vi "Elevator Controller.vi"(8 "error in (no error)":errorcluster, 11 "View Model":T1) -> (0 "error out":errorcluster)   [LabVIEW 2017]
doc: "Handles all elevator operations."
uses:
  View Model/Controls/View Model.ctl
  Error Handler/Controls/Error Model.ctl
  Error Handler/Controls/Error EventData.ctl
  Error Handler/Controls/Error Type.ctl
  Controls/Elevator Model.ctl
  Controls/Elevator Overhead.ctl
  Controls/Elevator States.ctl
  Controls/Elevator Location.ctl
  Controls/Elevator Command Event.ctl
  Controls/Elevator Commands.ctl
  Configuration/Controls/Configuration Model.ctl
  Configuration/Controls/Configuration Data.ctl
  View Model/Controls/Shared Model.ctl
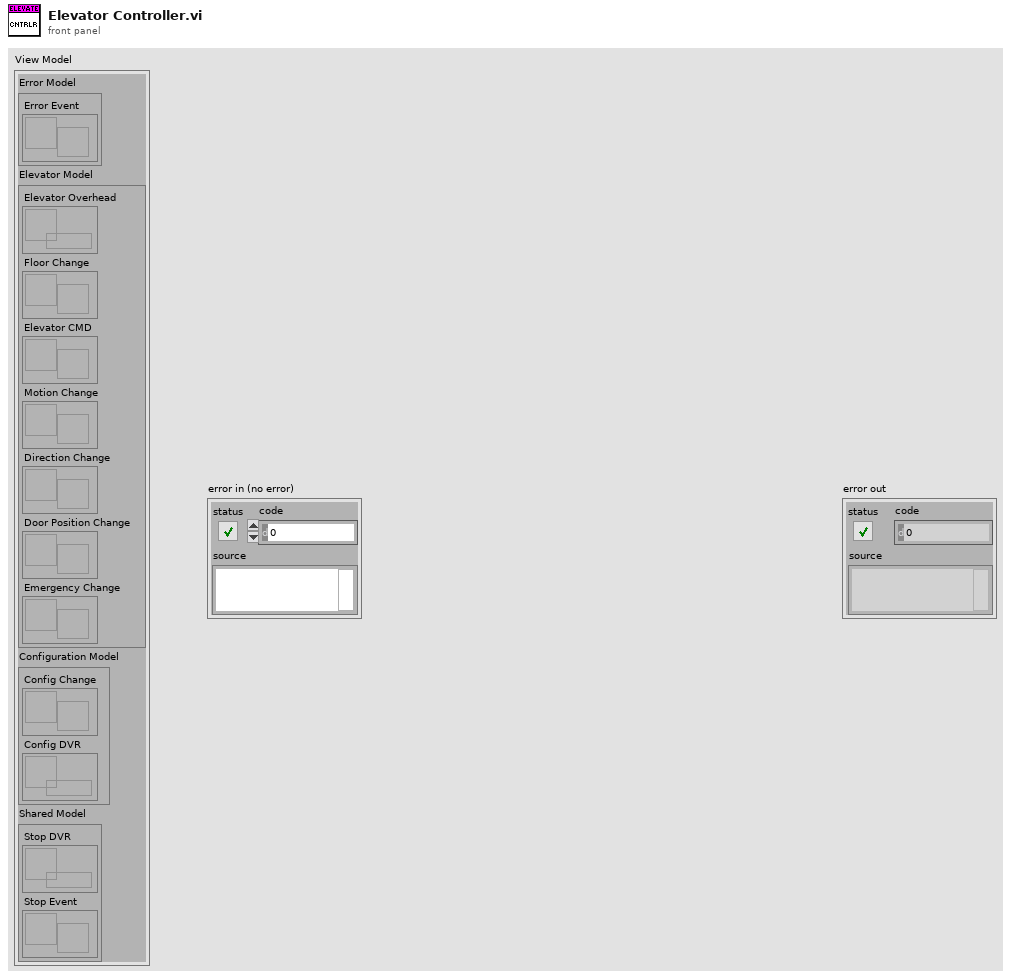
[diagram p1: front panel]
types:
  T1 = typedef "View Model.ctl" = cluster{"Error Model":T2, "Elevator Model":T3, "Configuration Model":T4, "Shared Model":T5}
  T2 = typedef "Error Model.ctl" = cluster{"Error Event":refnum<user-event>}
  T3 = typedef "Elevator Model.ctl" = cluster{"Elevator Overhead":refnum<data-value>, "Floor Change":refnum<user-event>, "Elevator CMD":refnum<user-event>, "Motion Change":refnum<user-event>, "Direction Change":refnum<user-event>, "Door Position Change":refnum<user-event>, "Emergency Change":refnum<user-event>}
  T4 = typedef "Configuration Model.ctl" = cluster{"Config Change":refnum<user-event>, "Config DVR":refnum<data-value>}
  T5 = typedef "Shared Model.ctl" = cluster{"Stop DVR":refnum<data-value>, "Stop Event":refnum<user-event>}
  T6 = typedef "Elevator Commands.ctl" = enum16{"Go Up", "Go Down", "Go to Floor", "Emergency", "Open Doors", "Close Doors"}
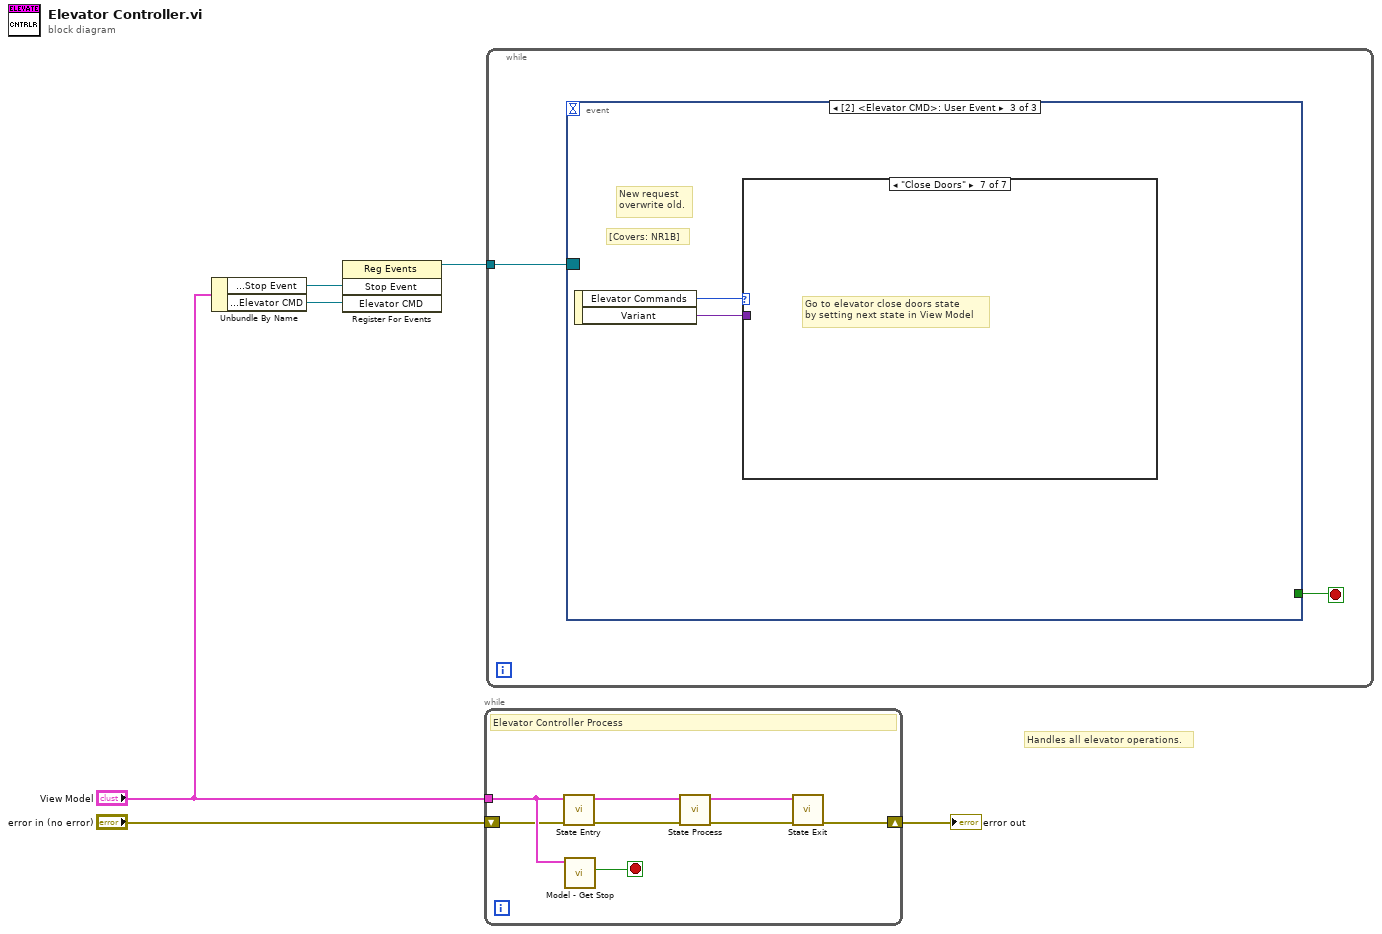
[diagram p0: block diagram]
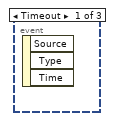
[diagram p2: hidden frame]
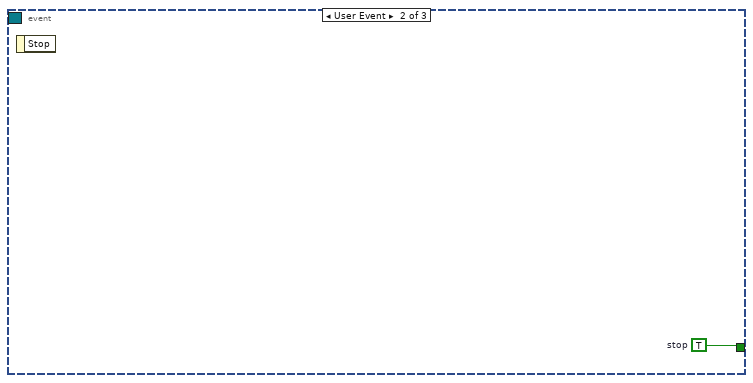
[diagram p3: hidden frame]
diagram:
  # "Handles all elevator operations."
  n1 = Unbundle By Name("View Model") -> ("Shared Model.Stop Event"=w6:refnum<user-event>, "Elevator Model.Elevator CMD"=w5:refnum<user-event>)
  n2 = register-events(w6, w5) -> (reference out=w4:refnum<event-registration>)  [unwired: 2 in, 1 out]
  n3 = while {
    tunnel: "View Model" -> [w9]
    shift-right: [w10] -> w1
    shift-left: "error in (no error)" -> [w8]
    stop <- w7 stop-if-true
    # "Elevator Controller Process"
    n4 = call "State Entry.vi"("error in (no error)"=w8, "View Model"=w9) -> ("error out"=w12:errorcluster, "View Model"=w14:T1)  [unwired: 8 in]
    n5 = call "Model - Get Stop.vi"("View Model"=w9) -> ("Stop?"=w7:bool)  [unwired: 8 in, 2 out]
    n6 = call "State Process.vi"("error in (no error)"=w12, "View Model"=w14) -> ("error out"=w11:errorcluster, "View Model"=w13:T1)  [unwired: 8 in]
    n7 = call "State Exit.vi"("error in (no error)"=w11, "View Model"=w13) -> ("error out"=w10:errorcluster)  [unwired: 8 in, 1 out]
  }
  "error out" <- w1
  n8 = while {
    tunnel: w4 -> [w16]
    stop <- w15 stop-if-true
    n9 = event shown="[2] <Elevator CMD>: User Event" {
      selector: w16 -> [_ _ _]
      dyn-events: _ -> [_ _ _]
      timeout: _ -> [_ _ _]
      tunnel: [_ w17 _] -> w15
      event Timeout {
        n10 = event-data() -> ()  [unwired: 1 in, 3 out]
      }
      event User Event {
        w17 = TRUE  # stop
        n11 = event-data() -> ()  [unwired: 1 in, 1 out]
      }
      event User Event {
        # "[Covers: NR1B]"
        # "New request \noverwrite old."
        n12 = event-data() -> ("Elevator Commands"=w19:T6, "Variant"=w18:variant)  [unwired: 1 in]
        n13 = case shown="\"Close Doors\"" w19 {
          tunnel: w18 -> [_ _ _ _ _ _ _]
          frame Default {
          }
          frame "Go Up" {
            # "[Covers: OC3A]"
            # "Go to elevator move up state\nby setting next state in View Model"
          }
          frame "Go Down" {
            # "Go to elevator move down state\nby setting next state in View Model"
          }
          frame "Go to Floor" {
            # "[Covers: WS3]"
            # "[Covers: WS2]"
            # "If on the first floor, set open doors to next state,\nelse set travel state"
            # "Go to elevator move up/down state\nby setting next state in View Model"
          }
          frame "Emergency" {
            # "Go to elevator emergency state\nby setting next state in View Model"
          }
          frame "Open Doors" {
            # "Go to elevator open doors state\nby setting next state in View Model"
          }
          frame "Close Doors" {
            # "Go to elevator close doors state\nby setting next state in View Model"
          }
        }
      }
    }
  }
